vi "Display_Filter.vi"(8 "Error in":errorcluster, 10 "Filter cluster":T1, 11 "Input data":cluster{dbl[], dbl[]}(graph)={array[3648 elements], array[3648 elements]}) -> (0 "Error out":errorcluster, 2 "Filter name":string, 3 "Output data":cluster{dbl[], dbl[]}[](graph))   [LabVIEW 2026]
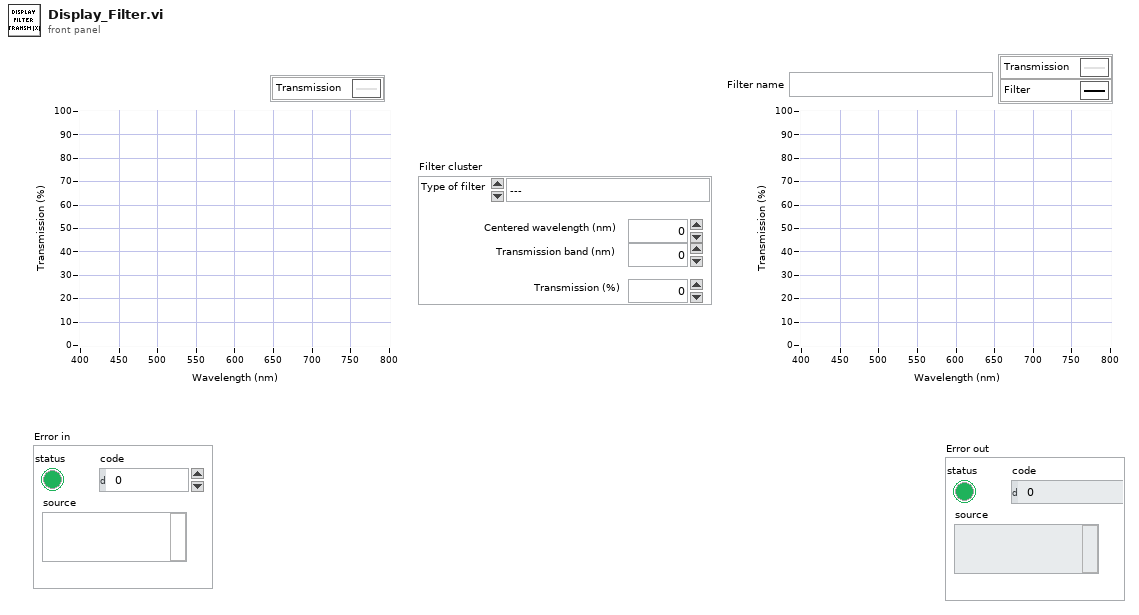
[diagram p1: front panel]
types:
  T1 = cluster{"Type of filter":enum16{"---", "Bandpass", "Longpass", "Shortpass"}, "Centered wavelength (nm)":dbl, "Transmission band (nm)":dbl, "Transmission (%)":dbl}
  T2 = enum16{"---", "Bandpass", "Longpass", "Shortpass"}
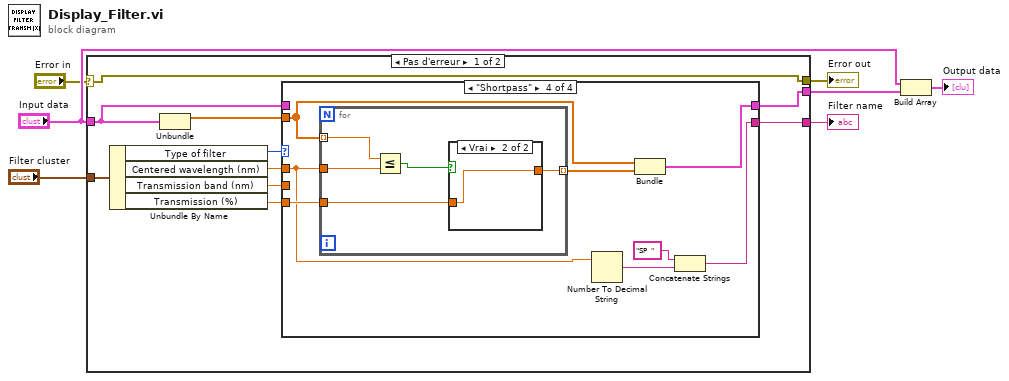
[diagram p0: block diagram]
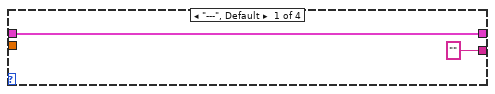
[diagram p2: hidden frame]
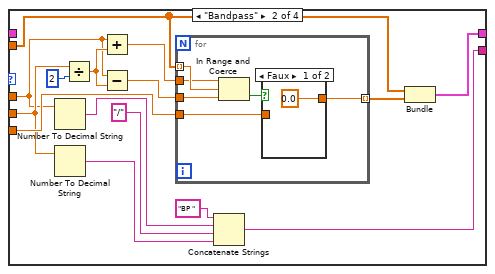
[diagram p3: hidden frame]
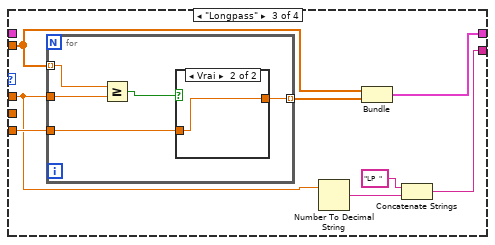
[diagram p5: hidden frame]
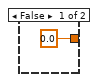
[diagram p6: hidden frame]
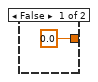
[diagram p7: hidden frame]
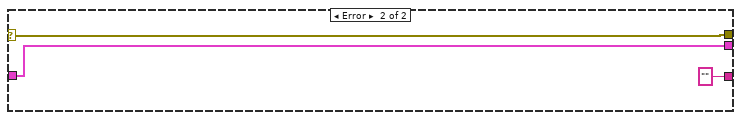
[diagram p8: hidden frame]
diagram:
  n1 = case shown="Pas d'erreur" "Error in" {
    selector: "Error in" -> [w13 w73]
    tunnel: "Input data" -> [w16 w74]
    tunnel: [w15 ""] -> w6
    tunnel: [w14 w74] -> w5
    tunnel: [w13 w73] -> w2
    tunnel: "Filter cluster" -> [w12 _]
    frame No Error {
      n2 = Unbundle By Name(w12) -> ("Type of filter"=w11:T2, "Centered wavelength (nm)"=w8:dbl, "Transmission band (nm)"=w10:dbl, "Transmission (%)"=w9:dbl)
      n3 = Unbundle(w16) -> (w17:dbl[])  [unwired: 1 out]
      n4 = case shown="\"Shortpass\"" w11 {
        tunnel: w17 -> [_ w29 w49 w64]
        tunnel: w9 -> [_ w30 w50 w65]
        tunnel: [w19 w27 w47 w62] -> w14
        tunnel: w16 -> [w19 _ _ _]
        tunnel: ["" w22 w44 w59] -> w15
        tunnel: w10 -> [_ w21 _ _]
        tunnel: w8 -> [_ w20 w43 w58]
        frame "---", Default {
        }
        frame "Bandpass" {
          n5 = Number To Decimal String(number=w20) -> (decimal integer string=w25:string)  [unwired: 1 in]
          n6 = Number To Decimal String(number=w21) -> (decimal integer string=w23:string)  [unwired: 1 in]
          n7 = Divide(x=w21, y=u8 2) -> (x/y=w33:dbl)
          n8 = Add(x=w20, y=w33) -> (x+y=w32:dbl)
          n9 = Subtract(x=w20, y=w33) -> (x-y=w31:dbl)
          n10 = for {
            tunnel: w29 -> [w40] mode=indexing
            tunnel: w32 -> [w39]
            tunnel: w31 -> [w38]
            tunnel: w30 -> [w36]
            tunnel: [w35] -> w28 mode=indexing
            n11 = In Range and Coerce(upper limit=w39, x=w40, lower limit=w38) -> (In Range?=w37:bool)  [unwired: 1 out]
            n12 = case shown="Faux" w37 {
              tunnel: w36 -> [_ w42]
              tunnel: [0.0 w42] -> w35
              frame False {
              }
              frame True {
              }
            }
          }
          n13 = Concatenate Strings("BP ", w25, "/", w23) -> (w22:string)
          n14 = Bundle(w29, w28) -> (w27:cluster{dbl[], dbl[]})  [unwired: 1 in]
        }
        frame "Longpass" {
          n15 = for {
            tunnel: w49 -> [w53] mode=indexing
            tunnel: w43 -> [w52]
            tunnel: w50 -> [w55]
            tunnel: [w54] -> w48 mode=indexing
            n16 = Greater Or Equal?(x=w53, y=w52) -> (x >= y?=w51:bool)
            n17 = case shown="Vrai" w51 {
              tunnel: w55 -> [_ w57]
              tunnel: [0.0 w57] -> w54
              frame False {
              }
              frame True {
              }
            }
          }
          n18 = Number To Decimal String(number=w43) -> (decimal integer string=w45:string)  [unwired: 1 in]
          n19 = Bundle(w49, w48) -> (w47:cluster{dbl[], dbl[]})  [unwired: 1 in]
          n20 = Concatenate Strings("LP  ", w45) -> (w44:string)
        }
        frame "Shortpass" {
          n21 = for {
            tunnel: w64 -> [w68] mode=indexing
            tunnel: w58 -> [w67]
            tunnel: w65 -> [w70]
            tunnel: [w69] -> w63 mode=indexing
            n22 = Less Or Equal?(x=w68, y=w67) -> (x <= y?=w66:bool)
            n23 = case shown="Vrai" w66 {
              tunnel: w70 -> [_ w72]
              tunnel: [0.0 w72] -> w69
              frame False {
              }
              frame True {
              }
            }
          }
          n24 = Number To Decimal String(number=w58) -> (decimal integer string=w60:string)  [unwired: 1 in]
          n25 = Bundle(w64, w63) -> (w62:cluster{dbl[], dbl[]})  [unwired: 1 in]
          n26 = Concatenate Strings("SP  ", w60) -> (w59:string)
        }
      }
    }
    frame Error {
    }
  }
  "Filter name" <- w6
  "Error out" <- w2
  n27 = Build Array("Input data", w5) -> (→"Output data":cluster{dbl[], dbl[]}[])
